vi "TestSCAN_MX5060.vi"(8 "errin":errorcluster) -> (0 "error out":errorcluster, 2 "Tableau 2":refnum<visa-resource-name>[](array[refnum]), 3 "Tableau":string[](array[string]))   [LabVIEW 2020]
doc: "Ce VI te sniff tout les équipement VISA qu'il détect et t'en fait une liste"
uses:
  <vilib>/Instr/_visa.llb/VISA Find Search Mode.ctl
  <vilib>/Instr/_visa.llb/VISA Configure Serial Port (Instr).vi
  <instrlib>/IT6000C/IT6000C.lvlib
  <vilib>/MakerHub/LINX/LMH-LINX.lvlib
  VG/ISOOCV.vi
  <vilib>/MakerHub/LINX/Public/Utilities/Open Serial.vi
panel:
  out "ISO OCV":string
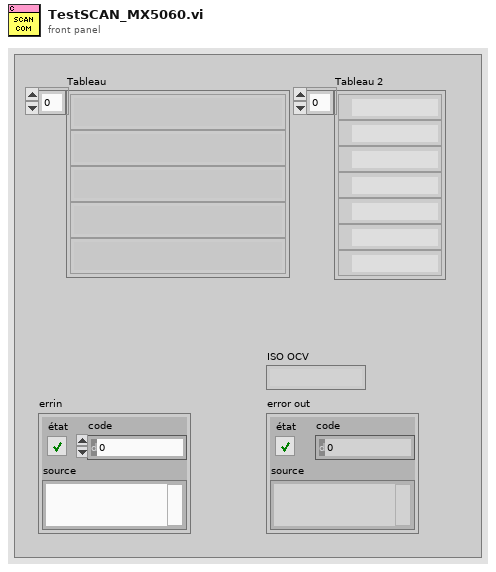
[diagram p1: front panel]
types:
  T1 = typedef "VISA Find Search Mode.ctl" = u32
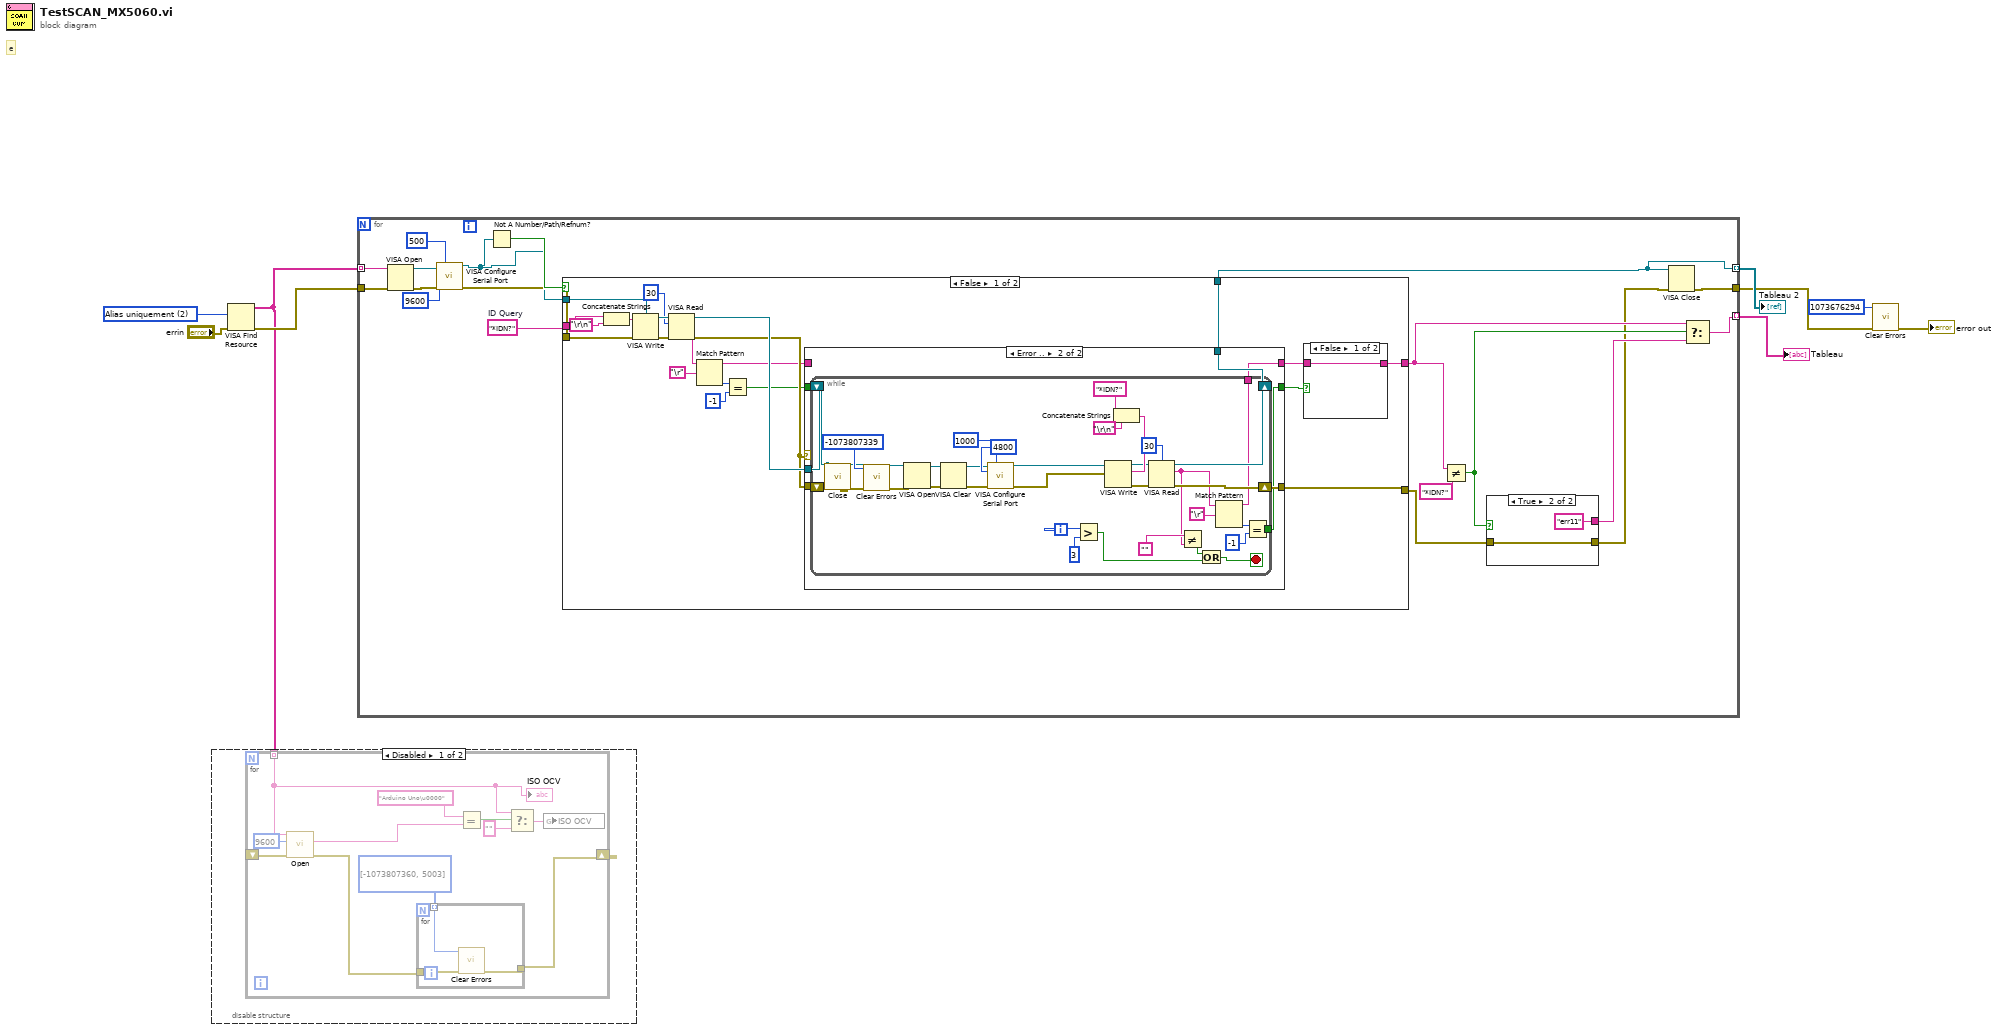
[diagram p0: block diagram]
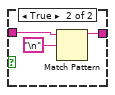
[diagram p4: hidden frame]
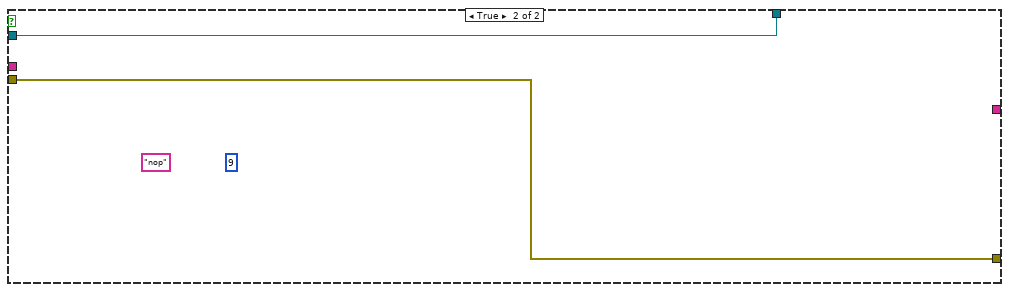
[diagram p5: hidden frame]
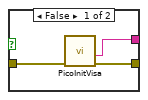
[diagram p6: hidden frame]
diagram:
  w6 = T1 2 items=["Noms canoniques uniquement"=0, "Alias uniquement"=2, "Inclure les alias correspondants"=3, "Inclure tous les alias"=4] ("Search Mode")
  # "e"
  n1 = VISA Find Resource(8:"errin", 10:w6) -> (0:w5:errorcluster, 3:w1:string[])  [unwired: 1 in, 1 out]
  n2 = disable-structure shown="Disabled" {
    disable-tunnel: w1 -> [w10 _]
    frame Disabled {
      n3 = for {
        tunnel: w10 -> [w12] mode=indexing
        shift-right: [w13] -> _
        shift-left: _ -> [w16]
        n4 = call-poly <vilib>:"Open.vi"("Error In"=w16, "Baud Rate Override"=u32 9600, "Serial Port"=w12) -> ("Error Out"=w18:errorcluster, "Device Name"=w19:string)  [unwired: 6 in, 1 out]
        n5 = for {
          tunnel: w18 -> [w24]
          tunnel: i32[] [-1073807360, 5003] -> [w23] mode=indexing
          tunnel: [w22] -> w13
          n6 = call <vilib>:"Clear Errors.vi"("error in (no error)"=w24, "specific error code to clear (0: all)"=w23) -> ("error out"=w22:errorcluster)  [unwired: 4 in, 1 out]
        }
        n7 = Equal?(x="Arduino Uno\u0000", y=w19) -> (x = y?=w21:bool)
        n8 = Select(t=w12, s=w21, f="") -> (s? t:f=w20:string)
        n9 = global write "ISOOCV.vi" "ISO OCV"(w20) -> ()
        "ISO OCV" <- w12
      }
    }
    frame Enabled {
    }
  }
  n10 = for {
    tunnel: w1 -> [w43] mode=indexing
    tunnel: [w36] -> w9 mode=indexing
    tunnel: [w25] -> w7 mode=indexing
    tunnel: w5 -> [w42]
    tunnel: [w26] -> w4
    w40 = "*IDN?"  # ID Query
    n11 = VISA Open(error in (no error)=w42, VISA resource name=w43) -> (VISA resource name=w31:refnum<visa-resource-name>, error out=w33:errorcluster)  [unwired: 3 in]
    n12 = call-poly "VISA Configure Serial Port"("VISA resource name"=w31, "timeout (10sec)"=u32 500, "baud rate (9600)"=u32 9600, "error in (no error)"=w33) -> ("VISA resource name out"=w29:refnum<visa-resource-name>, "error out"=w32:errorcluster)  [unwired: 10 in]
    n13 = Not A Number/Path/Refnum?(number/path/refnum=w29) -> (NaN/Path/Refnum?=w41:bool)
    n14 = case shown="False" w41 {
      tunnel: [w48 w113] -> w34
      tunnel: [w58 _] -> w35
      tunnel: w29 -> [w52 w112]
      tunnel: w40 -> [w57 _]
      tunnel: w32 -> [w55 w113]
      tunnel: [w49 w112] -> w25
      frame False {
        n15 = Concatenate Strings(w57, "\r\n") -> (w61:string)
        n16 = VISA Write(VISA resource name=w52, write buffer=w61, error in (no error)=w55) -> (VISA resource name out=w64:refnum<visa-resource-name>, error out=w63:errorcluster)  [unwired: 1 out]
        n17 = VISA Read(VISA resource name=w64, byte count=u32 30 ("nombre d'octets"), error in (no error)=w63) -> (VISA resource name out=w51:refnum<visa-resource-name>, read buffer=w54:string, error out=w50:errorcluster)  [unwired: 1 out]
        n18 = Match Pattern(string=w54, regular expression="\r") -> (before substring=w45:string, offset past match=w53:i32)  [unwired: 1 in, 2 out]
        n19 = Equal?(x=w53, y=-1) -> (x = y?=w46:bool)
        n20 = case shown="Error .." w50 {
          tunnel: w51 -> [w68 w69]
          tunnel: w50 -> [w67 w70]
          tunnel: [w68 w74] -> w49
          tunnel: [w67 w73] -> w48
          tunnel: [w66 w72] -> w47
          tunnel: w46 -> [w66 _]
          tunnel: w45 -> [w65 _]
          tunnel: [w65 w71] -> w44
          frame No Error {
          }
          frame Error {
            n21 = while {
              tunnel: [w97] -> w72
              tunnel: [w96] -> w71
              shift-right: [w101] -> w73
              shift-left: w70 -> [w92]
              shift-right: [w102] -> w74
              shift-left: w69 -> [w91]
              i -> [w81]
              stop <- w78 stop-if-true
              n22 = call <instrlib>:"Close.vi"("error in (no error)"=w92, "VISA resource name"=w91) -> ("error out"=w90:errorcluster)  [unwired: 9 in]
              n23 = call <vilib>:"Clear Errors.vi"("error in (no error)"=w90, "specific error code to clear (0: all)"=-1073807339) -> ("error out"=w94:errorcluster)  [unwired: 4 in, 1 out]
              n24 = VISA Open(error in (no error)=w94, VISA resource name=w91) -> (VISA resource name=w89:refnum<visa-resource-name>, error out=w88:errorcluster)  [unwired: 3 in]
              n25 = VISA Clear(VISA resource name=w89, error in (no error)=w88) -> (VISA resource name out=w86:refnum<visa-resource-name>, error out=w87:errorcluster)
              n26 = call-poly "VISA Configure Serial Port"("VISA resource name"=w86, "timeout (10sec)"=u32 1000, "baud rate (9600)"=u32 4800, "error in (no error)"=w87) -> ("VISA resource name out"=w77:refnum<visa-resource-name>, "error out"=w76:errorcluster)  [unwired: 10 in]
              n27 = Greater?(x=w81, y=3) -> (0:w79:bool)
              n28 = Concatenate Strings("*IDN?" ("chaîne"), "\r\n") -> (w105:string)
              n29 = VISA Write(VISA resource name=w77, write buffer=w105, error in (no error)=w76) -> (VISA resource name out=w85:refnum<visa-resource-name>, error out=w107:errorcluster)  [unwired: 1 out]
              n30 = VISA Read(VISA resource name=w85, byte count=u32 30 ("nombre d'octets"), error in (no error)=w107) -> (VISA resource name out=w102:refnum<visa-resource-name>, read buffer=w83:string, error out=w101:errorcluster)  [unwired: 1 out]
              n31 = Not Equal?(x="", y=w83) -> (x != y?=w82:bool)
              n32 = Or(x=w82, y=w79) -> (x .or. y?=w78:bool)
              n33 = Match Pattern(string=w83, regular expression="\r") -> (before substring=w96:string, offset past match=w98:i32)  [unwired: 1 in, 2 out]
              n34 = Equal?(x=w98, y=-1) -> (x = y?=w97:bool)
            }
          }
        }
        n35 = case shown="False" w47 {
          tunnel: [w108 w110] -> w58
          tunnel: w44 -> [w108 w109]
          frame False {
          }
          frame True {
            n36 = Match Pattern(string=w109, regular expression="\n") -> (before substring=w110:string)  [unwired: 1 in, 3 out]
          }
        }
      }
      frame True {
        (unwired) 9 ("offset past match")
        (unwired) "nop" ("read buffer")
      }
    }
    n37 = Not Equal?(x=w35, y="*IDN?") -> (x != y?=w38:bool)
    n38 = case shown="True" w38 {
      tunnel: [w116 w117] -> w27
      tunnel: [w115 "err11" ("data out")] -> w37
      tunnel: w34 -> [w114 w117]
      frame False {
        n39 = call "PicoInitVisa.vi"("errin"=w114) -> ("sortie d'erreur"=w116:errorcluster, "buffer de lecture 2"=w115:string)  [unwired: 7 in, 2 out]
      }
      frame True {
      }
    }
    n40 = VISA Close(VISA resource name=w25, error in (no error)=w27) -> (error out=w26:errorcluster)
    n41 = Select(t=w35, s=w38, f=w37) -> (s? t:f=w36:string)
  }
  "Tableau" <- w9
  "Tableau 2" <- w7
  n42 = call <vilib>:"Clear Errors.vi"("error in (no error)"=w4, "specific error code to clear (0: all)"=1073676294) -> ("error out"=→"error out":errorcluster)  [unwired: 4 in, 1 out]
